vi "Remove CR.vi"(5 "string":string) -> (2 "string out":string)   [LabVIEW 2019, in "ACSVcontrol-driver.lvlib"]
uses:
  ACSVcontrol-driver.lvlib
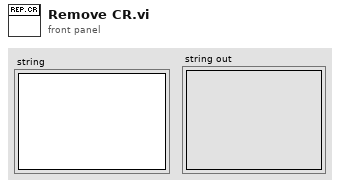
[diagram p1: front panel]
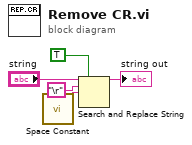
[diagram p0: block diagram]
diagram:
  n1 = call <vilib>:"Space Constant.vi"() -> ("String"=w2:string)
  n2 = Search and Replace String(replace all?=TRUE ("replace all? (F)"), input string="string", search string="\r", replace string=w2) -> (result string=→"string out":string)  [unwired: 4 in, 3 out]
